vi "Get Bucket Notification Configuration.vi"(8 "error in (no error)":errorcluster, 9 "Bucket":string) -> (0 "error out":errorcluster, 3 "NotificationConfiguration":T1)   [LabVIEW 2011, in "LV Interface for Amazon S3.lvlib"]
doc: "This operation <B>returns the notification configuration</B> of a bucket. If notifications are not enabled on the bucket, the operation returns an empty NotificatonConfiguration element. <B>You must be the bucket owner to read the notification configuration</B> of a bucket. The bucket owner can use a bucket policy to grant permission to other users to read this configuration with the s3:GetBucketNotification permission."
uses:
  LV Interface for Amazon S3.lvlib
  Typedefs/AMZ_S3_NotificationConfiguration.ctl
  Typedefs/AMZ_S3_TopicConfiguration.ctl
  Typedefs/AMZ_S3_Event.ctl
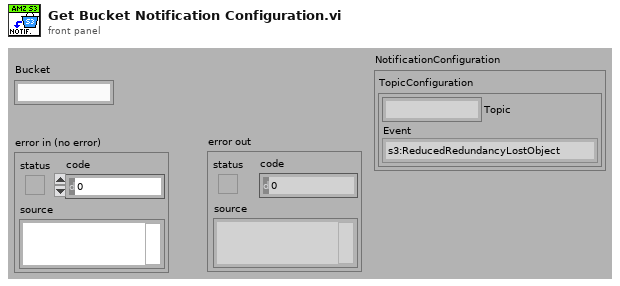
[diagram p1: front panel]
types:
  T1 = typedef "LV Interface for Amazon S3.lvlib/AMZ_S3_NotificationConfiguration.ctl" = cluster{"TopicConfiguration":T2}
  T2 = typedef "LV Interface for Amazon S3.lvlib/AMZ_S3_TopicConfiguration.ctl" = cluster{"Topic":string, "Event":T3}
  T3 = typedef "LV Interface for Amazon S3.lvlib/AMZ_S3_Event.ctl" = enum16{"s3:ReducedRedundancyLostObject"}
  T4 = typedef "LV Interface for Amazon S3.lvlib/AMZ_S3_Call Results.ctl" = enum16{"Success", "UndefinedError", "AccessDenied", "AccountProblem", "AmbiguousGrantByEmailAddress", "BadDigest", "BucketAlreadyExists", "BucketAlreadyOwnedByYou", "BucketNotEmpty", "CredentialsNotSupported", "CrossLocationLoggingProhibited", "EntityTooSmall", "EntityTooLarge", "ExpiredToken", "IllegalVersioningConfigurationException", "IncompleteBody", "IncorrectNumberOfFilesInPostRequest", "InlineDataTooLarge", "InternalError", "InvalidAccessKeyId", "InvalidAddressingHeader", "InvalidArgument", "InvalidBucketName", "InvalidDigest", "InvalidLocationConstraint", "InvalidPart", "InvalidPartOrder", "InvalidPayer", "InvalidPolicyDocument", "InvalidRange", "InvalidSecurity", "InvalidSOAPRequest", "InvalidStorageClass", "InvalidTargetBucketForLogging", "InvalidToken", "InvalidURI", "KeyTooLong", "MalformedACLError", "MalformedPOSTRequest", "MalformedXML", "MaxMessageLengthExceeded", "MaxPostPreDataLengthExceededError", "MetadataTooLarge", "MethodNotAllowed", "MissingAttachment", "MissingContentLength", "MissingRequestBodyError", "MissingSecurityElement", "MissingSecurityHeader", "NoLoggingStatusForKey", "NoSuchBucket", "NoSuchKey", "NoSuchUpload", "NoSuchVersion", "NotImplemented", "NotSignedUp", "OperationAborted", "PermanentRedirect", "PreconditionFailed", "Redirect", "RequestIsNotMultiPartContent", "RequestTimeout", "RequestTimeTooSkewed", "RequestTorrentOfBucketError", "SignatureDoesNotMatch", "SlowDown", "TemporaryRedirect", "TokenRefreshRequired", "TooManyBuckets", "UnexpectedContent", "UnresolvableGrantByEmailAddress", "UserKeyMustBeSpecified", "LabVIEWError"}
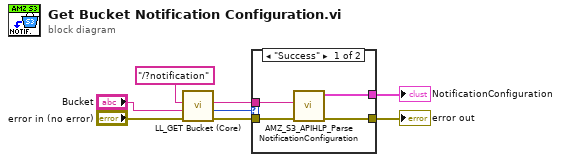
[diagram p0: block diagram]
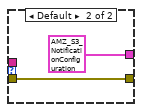
[diagram p2: hidden frame]
diagram:
  n1 = call "LL_GET Bucket (Core).vi"("error in (no error)"="error in (no error)", "Bucket"="Bucket", "Path and query string"="/?notification") -> ("error out"=w4:errorcluster, "Call Result"=w5:T4, "Response body"=w3:string)  [unwired: 5 in, 1 out]
  n2 = case shown="\"Success\"" w5 {
    tunnel: w4 -> [w12 w13]
    tunnel: w3 -> [w11 _]
    tunnel: [w10 T1 {"TopicConfiguration"={"Topic"="", "Event"=enum."s3:ReducedRedundancyLostObject"}} ("NotificationConfiguration")] -> w1
    tunnel: [w9 w13] -> w2
    frame "Success" {
      n3 = call "AMZ_S3_APIHLP_Parse NotificationConfiguration.vi"("error in (no error)"=w12, "Response body"=w11) -> ("error out"=w9:errorcluster, "NotificationConfiguration"=w10:T1)  [unwired: 8 in]
    }
    frame Default {
    }
  }
  "error out" <- w2
  "NotificationConfiguration" <- w1
